vi "Zeros and Extrema of f(x).vi"(0 "accuracy":dbl=1e-08 format="%.2e", 1 "step type":u16(ring) items=["fixed function", "modified function"], 2 "algorithm":u16(ring) items=["Ridders", "Newton Raphson"], 3 "start":dbl format="%.2f", 4 "end":dbl=1.0 format="%.2f", 5 "formula":string) -> (11 "error":i32, 13 "ticks":u32, 14 "Minima":dbl[](array[numeric]) format="%.2f", 15 "f(Minima)":dbl[](array[numeric]) format="%.2f", 16 "Zeros":dbl[](array[numeric]) format="%.2f", 17 "f(Zeros)":dbl[](array[numeric]) format="%.2f", 18 "Maxima":dbl[](array[numeric]) format="%.2f", 19 "f(Maxima)":dbl[](array[numeric]) format="%.2f")   [LabVIEW 2018, in "NI_Gmath.lvlib"]
doc: "Determines all zeros and extrema of a 1D function in a given interval."
uses:
  NI_Gmath.lvlib
panel:
  # "Example:\n\n accuracy: 1.0E-8\n step type: fixed function \n algorithm: Ridders\n start: -2.0\n end: 2.0\n formula: t^3-2*t+2"
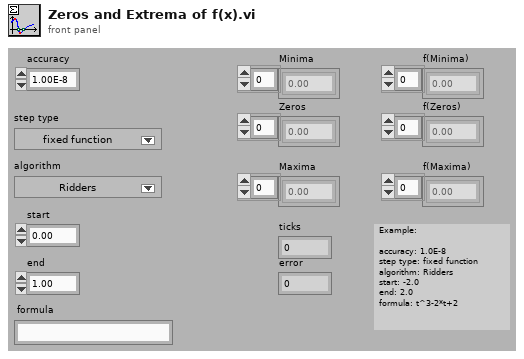
[diagram p1: front panel]
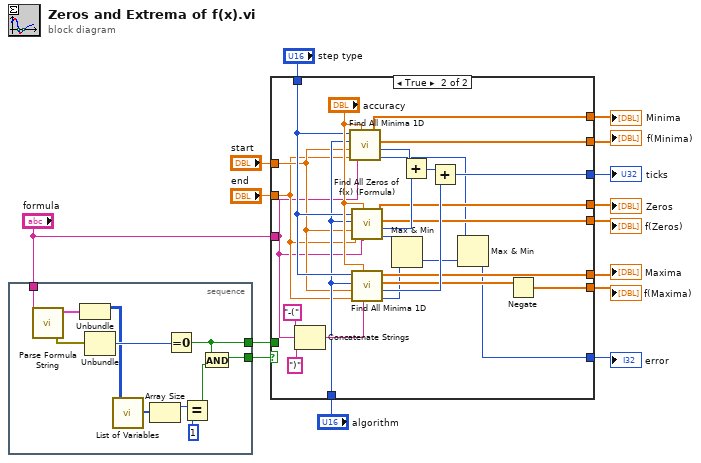
[diagram p0: block diagram]
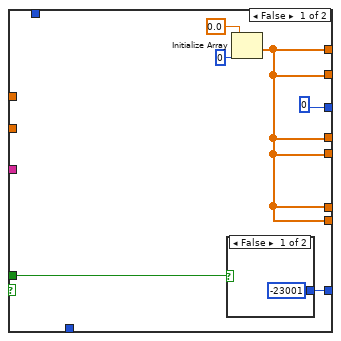
[diagram p2: hidden frame]
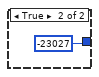
[diagram p3: hidden frame]
diagram:
  n1 = stacked-sequence {
    tunnel: [w26] -> w15
    tunnel: "formula" -> [w21]
    tunnel: [w18] -> w2
    frame #0 {
      n2 = call "Parse Formula String.vi"("formula"=w21) -> ("error out"=w20:errorcluster, "Parsed Formula"=w17:cluster{"Table":i32[][], "Y Values":dbl[]})  [unwired: 1 in]
      n3 = Unbundle(w17) -> ("Table"=w16:i32[][])  [unwired: 1 out]
      n4 = Unbundle(w20) -> ("code"=w19:i32)  [unwired: 2 out]
      n5 = call "List of Variables.vi"("Table"=w16) -> ("List of variables"=w22:i32[])
      n6 = Array Size(array=w22) -> (size(s)=w23:i32)
      n7 = Equal To 0?(x=w19) -> (x = 0?=w18:bool)
      n8 = Equal?(x=w23, y=1) -> (x = y?=w25:bool)
      n9 = And(x=w18, y=w25) -> (x .and. y?=w26:bool)
    }
  }
  n10 = case shown="True" w15 {
    tunnel: "step type" -> [_ w44]
    tunnel: "formula" -> [_ w40]
    tunnel: "start" -> [_ w42]
    tunnel: "end" -> [_ w41]
    tunnel: "algorithm" -> [_ w43]
    tunnel: [w29 w54] -> w9
    tunnel: [w29 w53] -> w8
    tunnel: [w29 w52] -> w7
    tunnel: [w29 w51] -> w6
    tunnel: [w29 w50] -> w5
    tunnel: [w29 w48] -> w4
    tunnel: [u32 0 w47] -> w3
    tunnel: w2 -> [w28 _]
    tunnel: [w27 w35] -> w1
    frame False {
      n11 = case shown="False" w28 {
        tunnel: [-23001 -23027] -> w27
        frame False {
        }
        frame True {
        }
      }
      n12 = Initialize Array(0.0, 0) -> (w29:dbl[])
    }
    frame True {
      n13 = Concatenate Strings("-(", w40, ")") -> (w46:string)
      n14 = call "Find All Minima 1D.vi"("formula"=w40, "accuracy"="accuracy", "end"=w41, "start"=w42, "algorithm"=w43, "step type"=w44) -> ("error"=w37:i32, "ticks"=w60:u32, "f(Minima)"=w53:dbl[], "Minima"=w54:dbl[])
      n15 = call "Find All Zeros of f(x) (Formula).vi"("formula"=w40, "accuracy"="accuracy", "end"=w41, "start"=w42, "algorithm"=w43, "step type"=w44) -> ("error"=w39:i32, "ticks"=w59:u32, "f(Zeros)"=w51:dbl[], "Zeros"=w52:dbl[])  [unwired: 2 in]
      n16 = call "Find All Minima 1D.vi"("formula"=w46, "accuracy"="accuracy", "end"=w41, "start"=w42, "algorithm"=w43, "step type"=w44) -> ("error"=w38:i32, "ticks"=w56:u32, "f(Minima)"=w49:dbl[], "Minima"=w50:dbl[])
      n17 = Max & Min(x=w39, y=w38) -> (min(x,y)=w36:i32)  [unwired: 1 out]
      n18 = Add(x=w60, y=w59) -> (x+y=w57:u32)
      n19 = Add(x=w57, y=w56) -> (x+y=w47:u32)
      n20 = Max & Min(x=w37, y=w36) -> (min(x,y)=w35:i32)  [unwired: 1 out]
      n21 = Negate(x=w49) -> (-x=w48:dbl[])
    }
  }
  "ticks" <- w3
  "Minima" <- w9
  "Zeros" <- w7
  "Maxima" <- w5
  "f(Zeros)" <- w6
  "f(Minima)" <- w8
  "f(Maxima)" <- w4
  "error" <- w1
